vi "CalcAngleCircle.vi"(1 "Vertical radius":dbl, 2 "Horizontal radius":dbl) -> (0 "Angle in degrees":dbl)   [LabVIEW 2009]
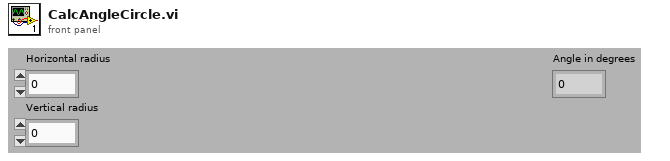
[diagram p1: front panel]
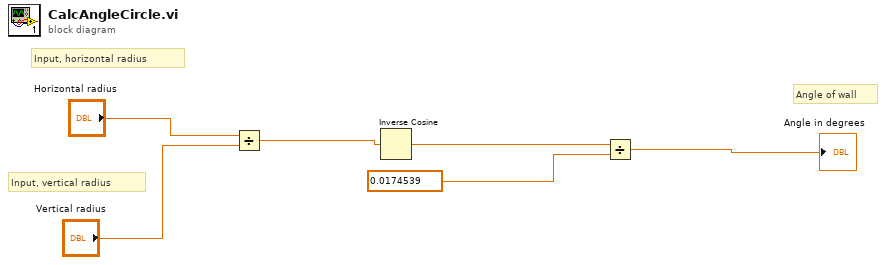
[diagram p0: block diagram]
diagram:
  # "Angle of wall"
  # "Input, vertical radius"
  # "Input, horizontal radius"
  n1 = Divide(x="Horizontal radius", y="Vertical radius") -> (x/y=w4:dbl)
  n2 = Inverse Cosine(1:w4) -> (0:w3:dbl)
  n3 = Divide(x=w3, y=0.0174539) -> (x/y=→"Angle in degrees":dbl)
